vi "2100_HV Load Test w_Telegram Write.vi"(0 "Semiconductor Module Context":T3, 1 "Reg0_State":string="State00", 2 "HSDIO_Pins":string[](array[string])=["CLK", "SDA"], 3 "Published_Data_ID":string="HV39_", 5 "HV_Load_Steps_uA":dbl[](array[numeric])=[0.0, 5.0, 8.0, 10.0] format="%#_6p", 7 "USID":T2 max=15, 9 "Reg_Address_Data":T1={"Address"=10, "Data"=133} {"Address" format="%.0x"}, 11 "error in (no error)":errorcluster, 12 "Num_Of_Telegrams":i32=10) -> (15 "error out":errorcluster)   [LabVIEW 2013]
uses:
  <vilib>/NI_TestStand_SemiconductorModule/NI_TestStand_Semiconductor_Module.lvlibp/PinMap/General/SemiconductorModuleContext.ctl
  Controls/USID.ctl
  Controls/Reg_Address_Data.ctl
  <instrlib>/niDCPower/nidcpower.llb/niDCPower Measurement Type.ctl
  <vilib>/NI_TestStand_SemiconductorModule/NI_TestStand_Semiconductor_Module.lvlibp/PinMap/DC Power/PinsToNIDCPowerSessions.vi
  <vilib>/NI_TestStand_SemiconductorModule/NI_TestStand_Semiconductor_Module.lvlibp/PinMap/Deprecated/PublishDataDoubleMultiplePinsSingleInstrument.vi
  <vilib>/NI_TestStand_SemiconductorModule/NI_TestStand_Semiconductor_Module.lvlibp
panel:
  out "current measurements":dbl[][](array[numeric]) format="%#_6p"
  out "voltage measurements":dbl[][](array[numeric])
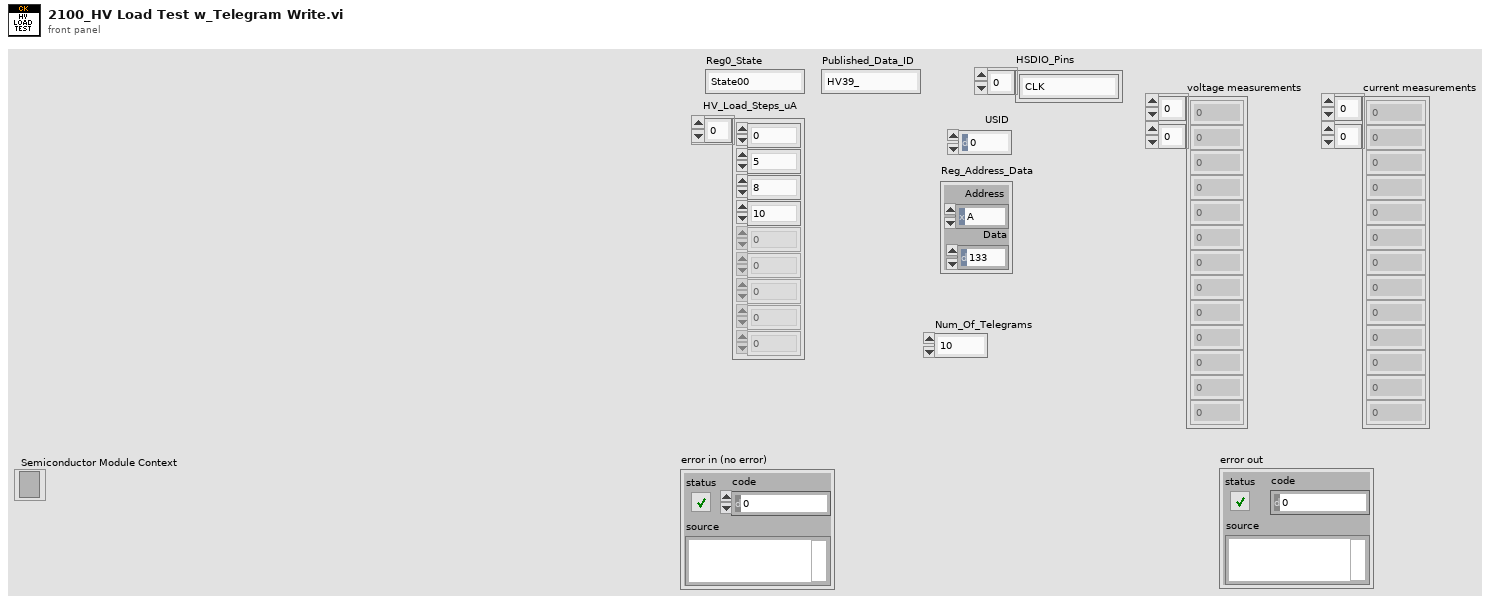
[diagram p1: front panel]
types:
  T1 = typedef "Reg_Address_Data.ctl" = cluster{"Address":u8, "Data":u8}
  T2 = typedef "USID.ctl" = u8
  T3 = typedef "NI_TestStand_Semiconductor_Module.lvlibp/SemiconductorModuleContext.ctl" = refnum<k7>
  T4 = typedef "niDCPower Measurement Type.ctl" = i32
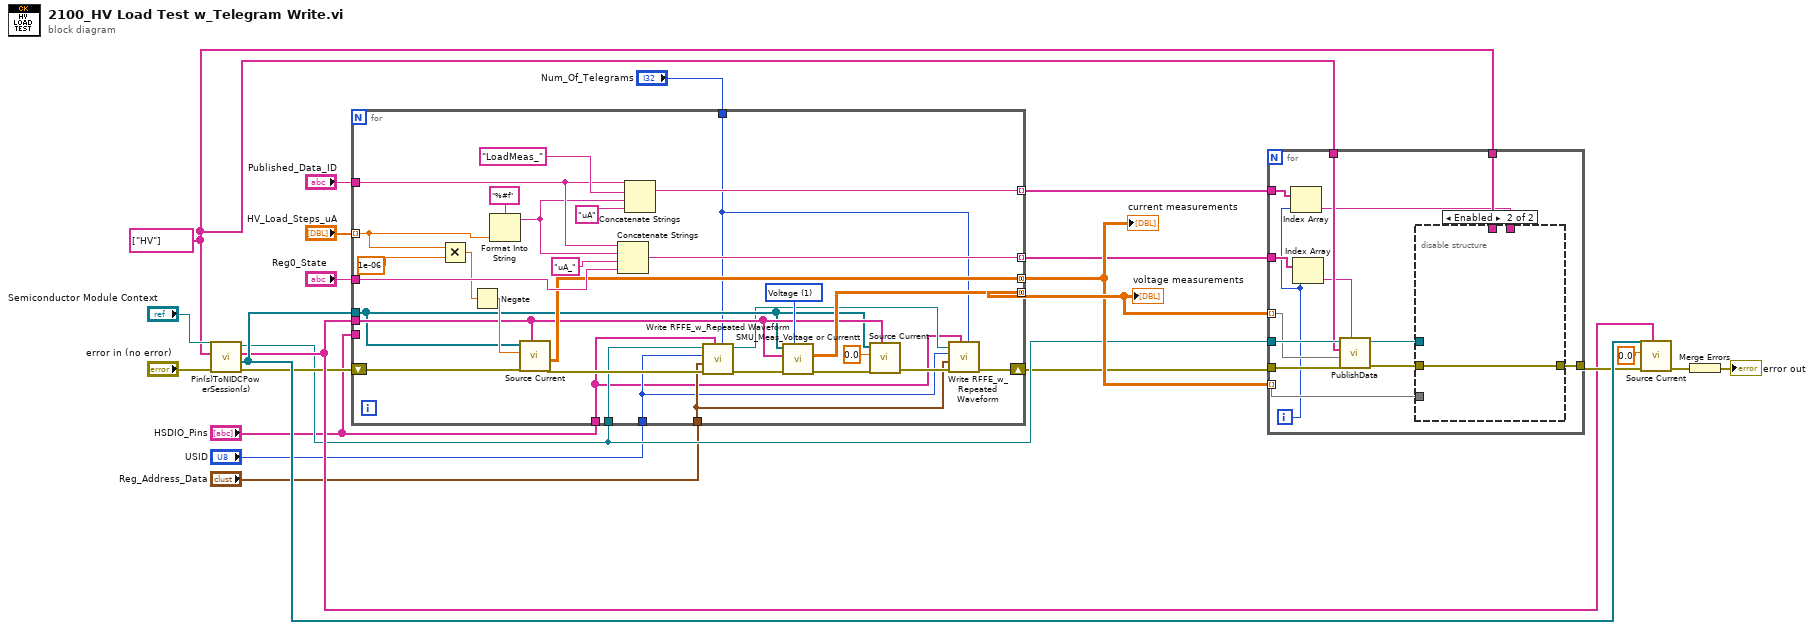
[diagram p0: block diagram]
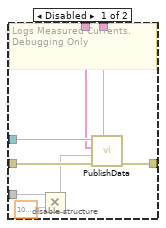
[diagram p2: hidden frame]
diagram:
  w15 = string[] ["HV"] ("Pins")
  n1 = call-poly <vilib>:"Pin(s)ToNIDCPowerSession(s).vi"("error in (no error)"="error in (no error)", "Pins"=w15, "Semiconductor Module Context"="Semiconductor Module Context") -> ("error out"=w8:errorcluster, "Instrument Sessions"=w22:refnum<k15>[], "Channel Lists"=w17:string[], "Semiconductor Module Context Out"=w6:T3)  [unwired: 4 in, 1 out]
  n2 = for {
    tunnel: w17 -> [w33]
    tunnel: "HV_Load_Steps_uA" -> [w42] mode=indexing
    tunnel: w22 -> [w32]
    shift-right: [w29] -> w5
    shift-left: w8 -> [w40]
    tunnel: "Published_Data_ID" -> [w48]
    tunnel: "Reg0_State" -> [w52]
    tunnel: [w35] -> w16 mode=concatenating
    tunnel: [w51] -> w11 mode=indexing
    tunnel: [w50] -> w14 mode=concatenating
    tunnel: [w47] -> w12 mode=indexing
    tunnel: w6 -> [w38]
    tunnel: "HSDIO_Pins" -> [_]
    tunnel: "HSDIO_Pins" -> [w25]
    tunnel: "USID" -> [w26]
    tunnel: "Reg_Address_Data" -> [w28]
    tunnel: "Num_Of_Telegrams" -> [w24]
    w37 = T4 1 items=["Current", "Voltage"] ("measurement type")
    n3 = Multiply(x=w42, y=1e-06) -> (x*y=w44:dbl)
    n4 = Negate(x=w44) -> (-x=w53:dbl)
    n5 = Format Into String(format string="%#f", w42) -> (resulting string=w41:string)  [unwired: 2 in, 1 out]
    n6 = call "Source Current.vi"("Channel Lists"=w33, "error in (no error)"=w40, "current level"=w53, "Instrument Sessions In"=w32) -> ("error out"=w39:errorcluster, "current measurements"=w50:dbl[][])  [unwired: 4 in, 2 out]
    n7 = Concatenate Strings(w48, w41, "uA_" ("string"), w52) -> (w51:string)
    n8 = Concatenate Strings(w48, "LoadMeas_" ("string"), w41, "uA" ("string")) -> (w47:string)
    n9 = call "Write RFFE_w_Repeated Waveform.vi"("Num_Of_Telegrams"=w24, "Pins"=w25, "error in (no error)"=w39, "Reg_Address_Data"=w28, "USID"=w26, "Semiconductor Module Context"=w38) -> ("error out"=w36:errorcluster, "Semiconductor Module Context Out"=w27:T3)  [unwired: 4 in]
    n10 = call "SMU_Meas_Voltage or Currentt.vi"("measurement type"=w37, "error in (no error)"=w36, "Channel Lists"=w33, "DCPower Sessions In"=w32) -> ("error out"=w34:errorcluster, "Measurement"=w35:dbl[][])  [unwired: 5 in, 1 out]
    n11 = call "Source Current.vi"("Channel Lists"=w33, "error in (no error)"=w34, "current level"=0.0, "Instrument Sessions In"=w32) -> ("error out"=w30:errorcluster)  [unwired: 4 in, 3 out]
    n12 = call "Write RFFE_w_Repeated Waveform.vi"("Num_Of_Telegrams"=w24, "Pins"=w25, "error in (no error)"=w30, "Reg_Address_Data"=w28, "USID"=w26, "Semiconductor Module Context"=w27) -> ("error out"=w29:errorcluster)  [unwired: 4 in, 1 out]
  }
  "voltage measurements" <- w16
  "current measurements" <- w14
  n13 = for {
    tunnel: w5 -> [w68]
    tunnel: [w64] -> w18
    tunnel: w6 -> [w67]
    tunnel: w16 -> [w66] mode=indexing
    tunnel: w15 -> [w65]
    tunnel: w15 -> [w61]
    tunnel: w14 -> [w60] mode=indexing
    tunnel: w11 -> [w59]
    tunnel: w12 -> [w58]
    i -> [w55]
    n14 = Index Array(array=w58, index=w55) -> (element=w57:string)
    n15 = Index Array(array=w59, index=w55) -> (element=w56:string)
    n16 = call-poly <vilib>:"PublishData.vi"("Measurement Id"=w56, "error in (no error)"=w68, "Data In"=w66, "Pins"=w65, "Semiconductor Module Context"=w67) -> ("error out"=w63:errorcluster, "Semiconductor Module Context Out"=w62:T3)  [unwired: 5 in]
    n17 = disable-structure shown="Enabled" {
      disable-tunnel: [w76 w77] -> w64
      disable-tunnel: w63 -> [w75 w77]
      disable-tunnel: w62 -> [w74 _]
      disable-tunnel: w61 -> [w73 _]
      disable-tunnel: w60 -> [w70 _]
      disable-tunnel: w57 -> [w69 _]
      frame Disabled {
        # "Logs Measured Currents.\nDebugging Only"
        n18 = Multiply(x=w70, y=1000000.0) -> (x*y=w72:dbl[])
        n19 = call-poly <vilib>:"PublishData.vi"("Measurement Id"=w69, "error in (no error)"=w75, "Data In"=w72, "Pins"=w73, "Semiconductor Module Context"=w74) -> ("error out"=w76:errorcluster)  [unwired: 5 in, 1 out]
      }
      frame Enabled {
      }
    }
  }
  n20 = call "Source Current.vi"("Channel Lists"=w17, "error in (no error)"=w18, "current level"=0.0, "Instrument Sessions In"=w22) -> ("error out"=w10:errorcluster)  [unwired: 4 in, 3 out]
  n21 = Merge Errors(w10) -> (→"error out":errorcluster)
